vi "Elevator.vi"(0 "Teleop Control":dbl) -> ()   [LabVIEW 2017]
uses:
  <vilib>/Rock Robotics/WPI/ThirdParty/Phoenix-LabVIEW/Motor Controller/Controls/CTRE_Phoenix_MotorControl_ControlMode.ctl
  Robot Global Data.vi
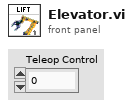
[diagram p1: front panel]
types:
  T1 = typedef "CTRE_Phoenix_MotorControl_ControlMode.ctl" = u16
  T2 = typedef "WPI_MotorControlDeviceRef.ctl" = cluster{"DeviceStatus":errorcluster, "Type":T3, "PWM":cluster{"PWM Channel":T4, "DeadBand":T5}, "CAN":cluster{"Device Number":u8, "SetOutput VI Ref":variant, "GetOutput VI Ref":variant, "Enable VI Ref":variant, "Disable VI Ref":variant, "Data":variant}, "Invert":bool, "DIO PWM":cluster{"PWM \"Enable\" Channel":T4, "DIOChannel":T6, "PWM Rate":dbl}}
  T3 = typedef "WPI_MotorControlType.ctl" = enum16{"PWM", "CAN", "DIO PWM"}
  T4 = typedef "FPGA_DIOPWMChannel.ctl" = enum8{"PWM 0", "PWM 1", "PWM 2", "PWM 3", "PWM 4", "PWM 5", "PWM 6", "PWM 7", "PWM 8", "PWM 9", "PWM MXP 0", "PWM MXP 1", "PWM MXP 2", "PWM MXP 3", "PWM MXP 4", "PWM MXP 5", "PWM MXP 6", "PWM MXP 7", "PWM MXP 8", "PWM MXP 9", "Invalid"}
  T5 = typedef "WPI_PWMDeadband.ctl" = cluster{"Name":string, "maxPositivePwm":i32, "minPositivePwm":i32, "centerPwm":i32, "maxNegativePwm":i32, "minNegativePwm":i32, "angularRange":u16}
  T6 = typedef "FPGA_DIOChannel.ctl" = enum8{"DIO 0", "DIO 1", "DIO 2", "DIO 3", "DIO 4", "DIO 5", "DIO 6", "DIO 7", "DIO 8", "DIO 9", "DIO MXP 0", "DIO MXP 1", "DIO MXP 2", "DIO MXP 3", "DIO MXP 4", "DIO MXP 5", "DIO MXP 6", "DIO MXP 7", "DIO MXP 8", "DIO MXP 9", "DIO MXP 10", "DIO MXP 11", "DIO MXP 12", "DIO MXP 13", "DIO MXP 14", "DIO MXP 15", "SPI Port CS1", "SPI Port CS2", "SPI Port CS3", "SPI Port MISO", "SPI Port MOSI", "Invalid"}
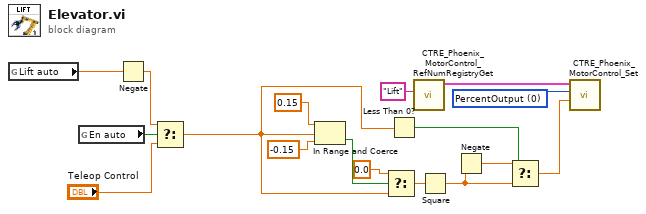
[diagram p0: block diagram]
diagram:
  w15 = T1 0 items=["PercentOutput"=0, "Position"=1, "Velocity"=2, "Current"=3, "Follower"=5, "MotionProfile"=6, "MotionMagic"=7, "MotionMagicArc"=8, "MotionProfileArc"=10, "Disabled"=15] ("Control Mode")
  n1 = global read "Robot Global Data.vi" "Lift auto"() -> (w2:dbl)
  n2 = global read "Robot Global Data.vi" "En auto"() -> (w13:bool)
  n3 = Negate(x=w2) -> (-x=w1:dbl)
  n4 = Select(t=w1, s=w13, f="Teleop Control") -> (s? t:f=w6:dbl)
  n5 = In Range and Coerce(upper limit=0.15, x=w6, lower limit=-0.15) -> (In Range?=w10:bool)  [unwired: 1 out]
  n6 = Select(t=0.0, s=w10, f=w6) -> (s? t:f=w8:dbl)
  n7 = Less Than 0?(x=w6) -> (x < 0?=w7:bool)
  n8 = call <vilib>:"CTRE_Phoenix_MotorControl_RefNumRegistryGet.vi"("refnum name"="Lift") -> ("PhoenixMotorControlDevRef"=w16:T2)  [unwired: 9 in, 1 out]
  n9 = Square(x=w8) -> (x^2=w4:dbl)
  n10 = Negate(x=w4) -> (-x=w5:dbl)
  n11 = Select(t=w5, s=w7, f=w4) -> (s? t:f=w3:dbl)
  n12 = call <vilib>:"CTRE_Phoenix_MotorControl_Set.vi"("Output"=w3, "Control Mode"=w15, "PhoenixMotorControlDevRef"=w16) -> ()  [unwired: 7 in, 2 out]
